vi "FTW-Image-Rectangle.vi"(1 "Fill Color":u32(colorbox)=16777216, 2 "Initial Picture":picture, 4 "Rectangle":T1 {"Left" format="%dpx"; "Top" format="%dpx"; "Right" format="%dpx"; "Bottom" format="%dpx"}, 5 "Border Color":u32(colorbox), 8 "Border Width":u8=1 format="%dpx") -> (7 "Picture":picture)   [LabVIEW 2014]
doc: "Draws a 1-, 4-, or 8-bit pixmap or a 24-bit RGB pixmap into a picture."
panel:
  # "Inputs"
  # "Outputs"
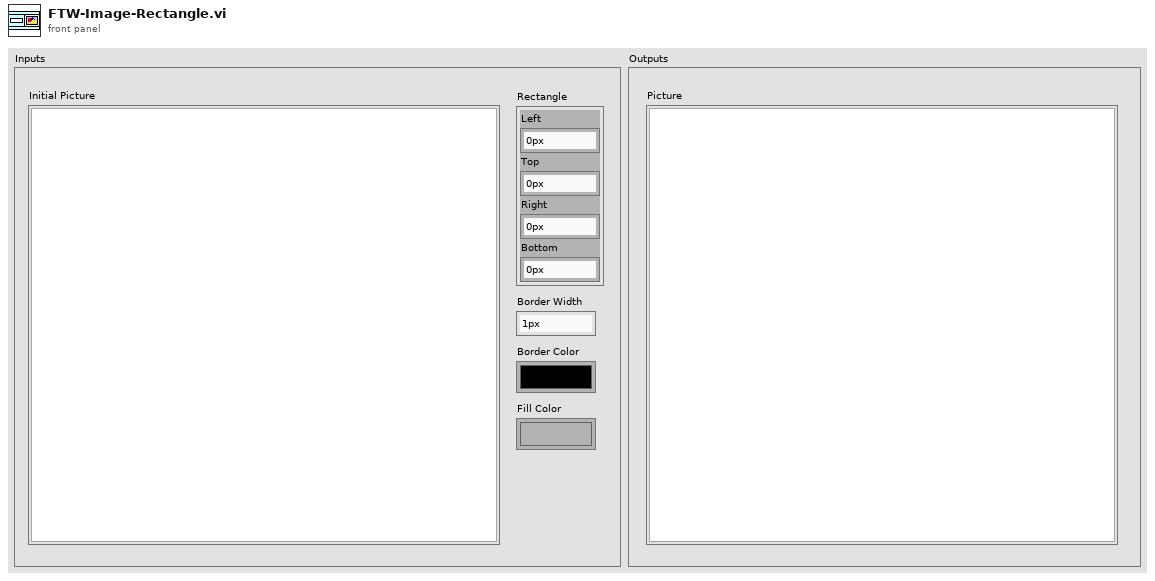
[diagram p1: front panel]
types:
  T1 = cluster{"Left":i32, "Top":i32, "Right":i32, "Bottom":i32}
  T2 = cluster{"Left":i16, "Top":i16, "Right":i16, "Bottom":i16}
  T3 = cluster{"opcode-Select Pen":i16, "size":i32, "PictPen ID":i32, "pen mask":i32, "Border Color":u32, "Border Width":i16, "Style":enum32{"Solid", "Dash", "Dot", "DashDot", "DashDotDot"}, "opcode-Frame Rect":i16, "size":i32, "top":i16, "left":i16, "bottom":i16, "right":i16}
  T4 = cluster{"opcode-Select Pen":i16, "size":i32, "PictPen ID":i32, "pen mask":i32, "Fill Color":u32, "Border Width (unused)":i16, "Style":enum32{"Solid", "Dash", "Dot", "DashDot", "DashDotDot"}, "opcode-Paint Rect":i16, "size":i32, "top":i16, "left":i16, "bottom":i16, "right":i16, "opcode-Select Pen 2":i16, "size 2":i32, "PictPen ID 2":i32, "pen mask 2":i32, "Border Color":u32, "Border Width":i16, "Style 2":enum32{"Solid", "Dash", "Dot", "DashDot", "DashDotDot"}, "opcode-Frame Rect 2":i16, "size":i32, "top2":i16, "left2":i16, "bottom2":i16, "right2":i16}
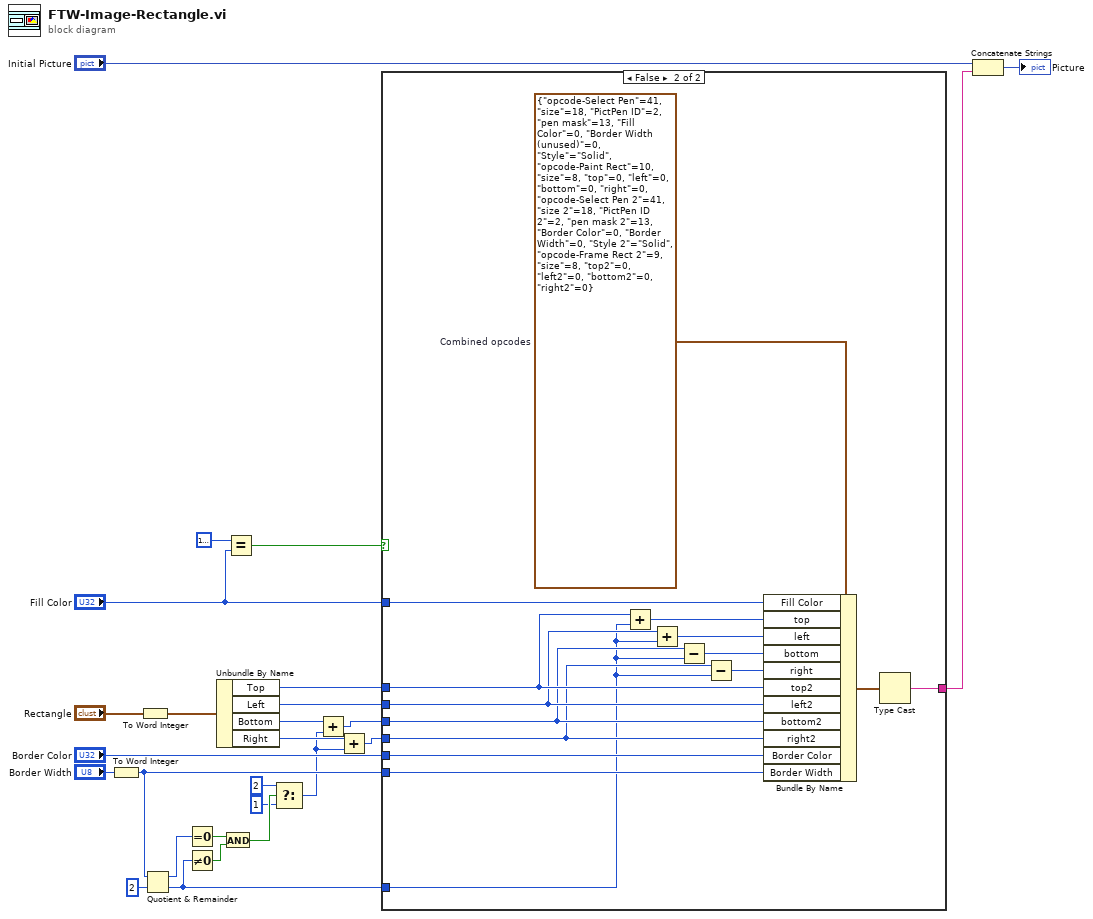
[diagram p0: block diagram]
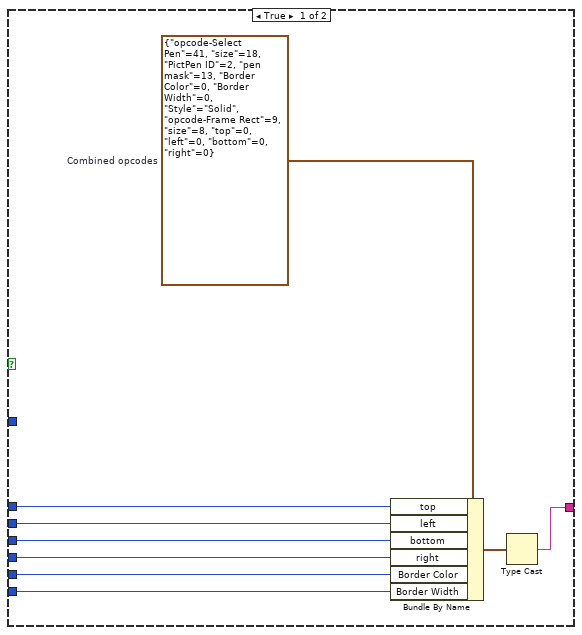
[diagram p2: hidden frame]
diagram:
  n1 = To Word Integer(number="Border Width") -> (16bit integer=w8:i16)
  n2 = To Word Integer(number="Rectangle") -> (16bit integer=w1:T2)
  n3 = Quotient & Remainder(x=w8, y=i16 2) -> (x-y*floor(x/y)=w10:i16, floor(x/y)=w2:i16)
  n4 = Equal To 0?(x=w10) -> (x = 0?=w11:bool)
  n5 = Not Equal To 0?(x=w2) -> (x != 0?=w9:bool)
  n6 = Unbundle By Name(w1) -> ("Top"=w21:i16, "Left"=w20:i16, "Bottom"=w22:i16, "Right"=w23:i16)
  n7 = And(x=w11, y=w9) -> (x .and. y?=w14:bool)
  n8 = Equal?(x=u32 16777216 ("Fill Color"), y="Fill Color") -> (x = y?=w4:bool)
  n9 = Select(t=i16 2, s=w14, f=i16 1) -> (s? t:f=w7:i16)
  n10 = Add(x=w22, y=w7) -> (x+y=w6:i16)
  n11 = Add(x=w23, y=w7) -> (x+y=w5:i16)
  n12 = case shown="False" w4 {
    tunnel: w21 -> [w35 w44]
    tunnel: w20 -> [w34 w42]
    tunnel: "Border Color" -> [w33 w50]
    tunnel: [w32 w49] -> w16
    tunnel: w8 -> [w31 w48]
    tunnel: w6 -> [w29 w40]
    tunnel: w5 -> [w28 w38]
    tunnel: "Fill Color" -> [_ w45]
    tunnel: w2 -> [_ w36]
    frame True {
      w30 = T3 {"opcode-Select Pen"=41, "size"=18, "PictPen ID"=2, "pen mask"=13, "Border Color"=0, "Border Width"=0, "Style"=enum."Solid", "opcode-Frame Rect"=9, "size"=8, "top"=0, "left"=0, "bottom"=0, "right"=0}  # Combined opcodes
      n13 = Bundle By Name(cluster=w30, "top"=w35, "left"=w34, "bottom"=w29, "right"=w28, "Border Color"=w33, "Border Width"=w31) -> (w27:T3)
      n14 = Type Cast(x=w27) -> (*(type *) &x=w32:string)  [unwired: 1 in]
    }
    frame False {
      w47 = T4 {"opcode-Select Pen"=41, "size"=18, "PictPen ID"=2, "pen mask"=13, "Fill Color"=0, "Border Width (unused)"=0, "Style"=enum."Solid", "opcode-Paint Rect"=10, "size"=8, "top"=0, "left"=0, "bottom"=0, "right"=0, "opcode-Select Pen 2"=41, "size 2"=18, "PictPen ID 2"=2, "pen mask 2"=13, "Border Color"=0, "Border Width"=0, "Style 2"=enum."Solid", "opcode-Frame Rect 2"=9, "size"=8, "top2"=0, "left2"=0, "bottom2"=0, "right2"=0}  # Combined opcodes
      n15 = Add(x=w44, y=w36) -> (x+y=w43:i16)
      n16 = Add(x=w42, y=w36) -> (x+y=w41:i16)
      n17 = Subtract(x=w40, y=w36) -> (x-y=w39:i16)
      n18 = Subtract(x=w38, y=w36) -> (x-y=w37:i16)
      n19 = Bundle By Name(cluster=w47, "Fill Color"=w45, "top"=w43, "left"=w41, "bottom"=w39, "right"=w37, "top2"=w44, "left2"=w42, "bottom2"=w40, "right2"=w38, "Border Color"=w50, "Border Width"=w48) -> (w46:T4)
      n20 = Type Cast(x=w46) -> (*(type *) &x=w49:string)  [unwired: 1 in]
    }
  }
  n21 = Concatenate Strings("Initial Picture", w16) -> (→"Picture":picture)
